vi "Write.vi"(7 "I2C Channel":u8, 8 "Error In":errorcluster, 10 "Time Stamp":timestamp, 11 "LINX Resource":T1) -> (0 "Error Out":errorcluster, 3 "LINX Resource":T1)   [LabVIEW 2011, in "LMH-LINX.lvlib" / "DS1307.lvlib"]
uses:
  DS1307.lvlib
  Private/Type Defs/LINX Ref.ctl
  Private/Type Defs/Platform.ctl
  Private/Type Defs/Interface.ctl
  Private/Device/Type Defs/LINX Device Config.ctl
  Private/Device/Type Defs/TCP Config.ctl
  Private/Device/Type Defs/Channels.ctl
  LMH-LINX.lvlib
  <vilib>/MakerHub/Toolbox/LMH-Toolbox.lvlib
  Private/Device/Device.lvlib
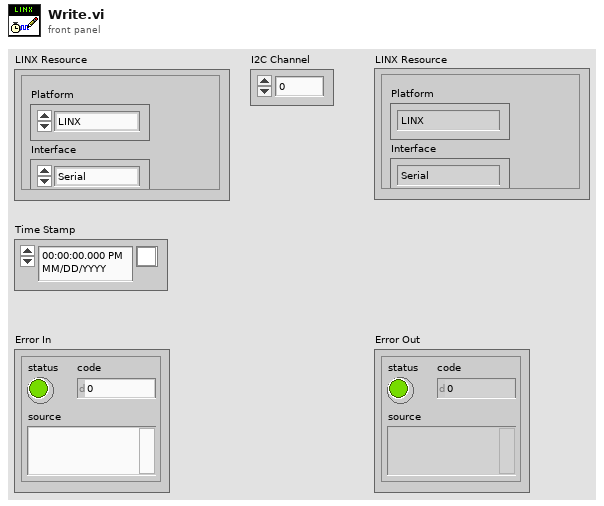
[diagram p1: front panel]
types:
  T1 = typedef "LMH-LINX.lvlib/LINX Ref.ctl" = cluster{"Platform":T2, "Interface":T3, "LINX Device Config":T4}
  T2 = typedef "LMH-LINX.lvlib/Platform.ctl" = enum16{"LINX", "myRIO"}
  T3 = typedef "LMH-LINX.lvlib/Interface.ctl" = enum16{"Serial", "TCP"}
  T4 = typedef "LMH-LINX.lvlib/Device.lvlib/LINX Device Config.ctl" = cluster{"Interface":T3, "COM Port":refnum<visa-resource-name>, "TCP Configuration":T5, "Device Family":u8, "Device ID":u8, "Device Name":string, "TCP Ref":refnum<k5>, "Channels":T6}
  T5 = typedef "LMH-LINX.lvlib/Device.lvlib/TCP Config.ctl" = cluster{"IP Address":string, "Port":u16}
  T6 = typedef "LMH-LINX.lvlib/Channels.ctl" = cluster{"DI":u8[], "DO":u8[], "AI":u8[], "AO":u8[], "PWM":u8[], "QE":u8[], "UART":u8[], "I2C 2":u8[], "SPI":u8[], "CAN":u8[], "Servo":u8[], "AI Ref (V)":dbl, "AO Ref (V)":dbl, "AO Resolution (Bits)":u8}
  T7 = typedef "LVDateTimeRec.ctl" = cluster{"fractional second":dbl, "second":i32, "minute":i32, "hour":i32, "day of month":i32, "month":i32, "year":i32, "day of week":i32, "day of year":i32, "DST":i32}
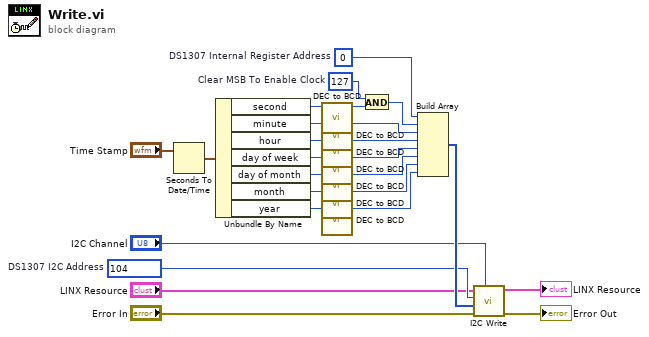
[diagram p0: block diagram]
diagram:
  w6 = u8 104  # DS1307 I2C Address
  w15 = u8 0  # DS1307 Internal Register Address
  w16 = u8 127  # Clear MSB To Enable Clock
  n1 = Seconds To Date/Time(time stamp (now)="Time Stamp") -> (date time rec=w25:T7)  [unwired: 1 in]
  n2 = Unbundle By Name(w25) -> ("second"=w24:i32, "minute"=w23:i32, "hour"=w22:i32, "day of week"=w21:i32, "day of month"=w20:i32, "month"=w19:i32, "year"=w18:i32)
  n3 = call <vilib>:"DEC to BCD.vi"("DEC"=w24) -> ("BCD"=w17:u8)  [unwired: 10 in]
  n4 = call <vilib>:"DEC to BCD.vi"("DEC"=w23) -> ("BCD"=w13:u8)  [unwired: 10 in]
  n5 = call <vilib>:"DEC to BCD.vi"("DEC"=w22) -> ("BCD"=w12:u8)  [unwired: 10 in]
  n6 = call <vilib>:"DEC to BCD.vi"("DEC"=w21) -> ("BCD"=w11:u8)  [unwired: 10 in]
  n7 = call <vilib>:"DEC to BCD.vi"("DEC"=w20) -> ("BCD"=w10:u8)  [unwired: 10 in]
  n8 = call <vilib>:"DEC to BCD.vi"("DEC"=w19) -> ("BCD"=w9:u8)  [unwired: 10 in]
  n9 = call <vilib>:"DEC to BCD.vi"("DEC"=w18) -> ("BCD"=w8:u8)  [unwired: 10 in]
  n10 = And(x=w16, y=w17) -> (x .and. y?=w14:u8)
  n11 = Build Array(w15, w14, w13, w12, w11, w10, w9, w8) -> (w7:u8[])
  n12 = call "I2C Write.vi"("I2C Channel"="I2C Channel", "Error In"="Error In", "Data"=w7, "I2C Slave Address (0)"=w6, "LINX Resource"="LINX Resource") -> ("Error Out"=→"Error Out":errorcluster, "LINX Resource"=→"LINX Resource":T1)  [unwired: 5 in]
